vi "Find Installs.vi"(8 "error in":errorcluster, 11 "TSDiscovery Mock in":refnum<class "TSDiscovery Mock.lvclass">) -> (0 "error out":errorcluster, 3 "TSInstalls Out":T1[](array[typedef]))   [LabVIEW 2025, in "TSDiscovery Mock.lvclass"]
doc: "FindInstalls.vi returns a predefined set of TSInstall instances and does not perform any real system discovery.\n\nIn this mock implementation, the method simulates a system with the following TestStand installations:\n- TestStand 2025 (64-bit)\n- TestStand 2025 (32-bit)\n- TestStand 2023 (64-bit)\n\nThe returned data is static and fully deterministic, enabling repeatable unit and component tests that are independent of the host system. This implementation is intended solely for testing and validation purposes and must not be used in production code."
uses:
  TSDiscovery Mock.lvclass
  Type Definitions/TSInstall--cluster.ctl
  Type Definitions/Architecture--enum.ctl
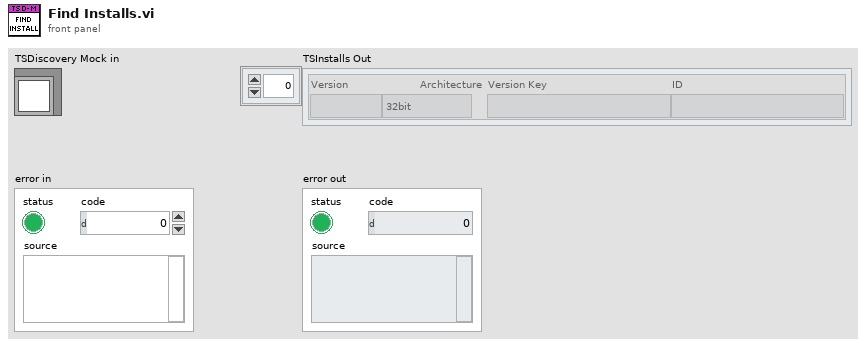
[diagram p1: front panel]
types:
  T1 = typedef "TSInstall--cluster.ctl" = cluster{"Version":string, "Architecture":T2, "Version Key":string, "ID":string}
  T2 = typedef "Architecture--enum.ctl" = enum16{"32bit", "64bit"}
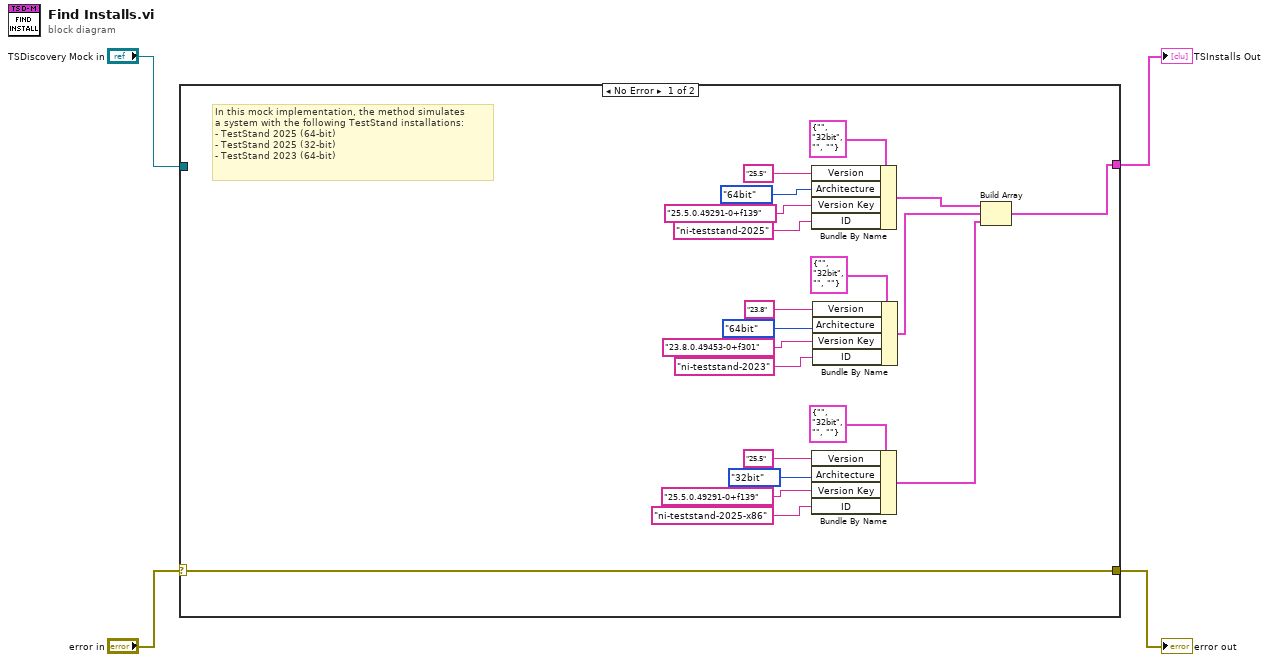
[diagram p0: block diagram]
diagram:
  n1 = case shown="No Error" "error in" {
    selector: "error in" -> [w7 w25]
    tunnel: [w7 w25] -> w3
    tunnel: "TSDiscovery Mock in" -> [_ _]
    tunnel: [w8 _] -> w1
    frame No Error {
      # "In this mock implementation, the method simulates \na system with the following TestStand installations:\n- TestStand 2025 (64-bit)\n- TestStand 2025 (32-bit)\n- TestStand 2023 (64-bit)"
      n2 = Bundle By Name(cluster=T1 {"Version"="", "Architecture"=enum."32bit", "Version Key"="", "ID"=""} ("TSInstalls Out"), "Version"="25.5", "Architecture"=Architecture--enum."64bit", "Version Key"="25.5.0.49291-0+f139", "ID"="ni-teststand-2025") -> (w11:T1)
      n3 = Bundle By Name(cluster=T1 {"Version"="", "Architecture"=enum."32bit", "Version Key"="", "ID"=""} ("TSInstalls Out"), "Version"="25.5", "Architecture"=Architecture--enum."32bit", "Version Key"="25.5.0.49291-0+f139", "ID"="ni-teststand-2025-x86") -> (w10:T1)
      n4 = Bundle By Name(cluster=T1 {"Version"="", "Architecture"=enum."32bit", "Version Key"="", "ID"=""} ("TSInstalls Out"), "Version"="23.8", "Architecture"=Architecture--enum."64bit", "Version Key"="23.8.0.49453-0+f301", "ID"="ni-teststand-2023") -> (w9:T1)
      n5 = Build Array(w11, w9, w10) -> (w8:T1[])
    }
    frame Error {
      # "Pass error without further action"
    }
  }
  "TSInstalls Out" <- w1
  "error out" <- w3
